vi "Read Binary Config.vi"(4 "Class Name is Included":bool, 6 "byte order (0:big-endian, network order)":T1(ring), 8 "error in (no error)":errorcluster, 10 "Binary":string, 11 "Const_Bool in":refnum<class "Const_Bool.lvclass">) -> (0 "error out":errorcluster, 2 "Remaining":string, 3 "Const_Bool out":refnum<class "Const_Bool.lvclass">)   [LabVIEW 2021, in "Const_Bool.lvclass"]
uses:
  Const_Bool.lvclass
  Const_Bool.lvclass/Const_Bool.ctl
  Abs_Types/Boolean/Abs_Boolean.lvclass
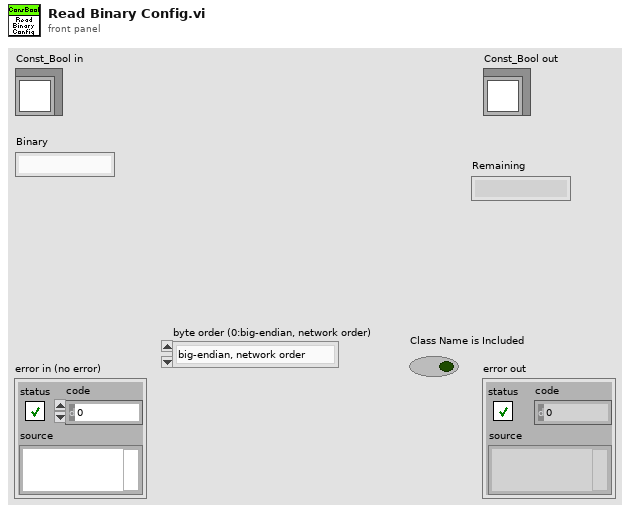
[diagram p1: front panel]
types:
  T1 = enum16{"big-endian, network order", "native, host order", "little-endian"}
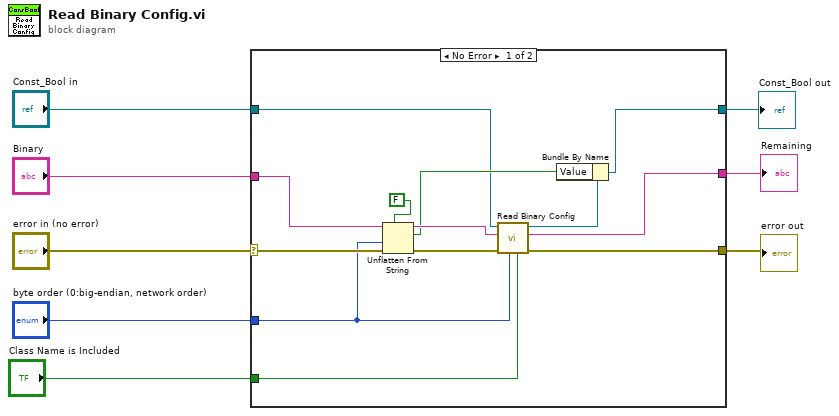
[diagram p0: block diagram]
diagram:
  n1 = case shown="No Error" "error in (no error)" {
    selector: "error in (no error)" -> [w19 w23]
    tunnel: [w14 w23] -> w6
    tunnel: [w11 w24] -> w3
    tunnel: "byte order (0:big-endian, network order)" -> [w16 _]
    tunnel: "Const_Bool in" -> [w13 w24]
    tunnel: "Binary" -> [w21 w22]
    tunnel: "Class Name is Included" -> [w10 _]
    tunnel: [w9 w22] -> w1
    frame No Error {
      n2 = Unflatten From String(type=FALSE, binary string=w21, byte order (0:big-endian, network order)=w16, error in (no error)=w19) -> (rest of the binary string=w20:string, value=w17:bool, error out=w18:errorcluster)  [unwired: 1 in]
      n3 = call-parent "Read Binary Config.vi"("Class Name is Included"=w10, "byte order (0:big-endian, network order)"=w16, "error in (no error)"=w18, "Binary"=w20, "Abs_Type in"=w13) -> ("error out"=w14:errorcluster, "Remaining"=w9:string, "Abs_Type out"=w12:refnum<class "Const_Bool.lvclass">)  [unwired: 4 in]
      n4 = Bundle By Name(cluster=w12, "Value"=w17) -> (w11:refnum<class "Const_Bool.lvclass">)
    }
    frame Error {
    }
  }
  "error out" <- w6
  "Const_Bool out" <- w3
  "Remaining" <- w1
